vi "使用范例_单行数据存储A.vi"() -> ()   [LabVIEW 2020]
panel:
  in  "文件头（最后一个字符是换行）":string="Current Voltage\nI V\n"
  in  "存储路径":path=path "D:/"
  in  "其他说明信息":string="300K_1000Oe"
  in  "测试项目":string="IVcurve"
  in  "样品名称":string="deviceUnderTest"
  in  "是否添加时间？":bool=TRUE
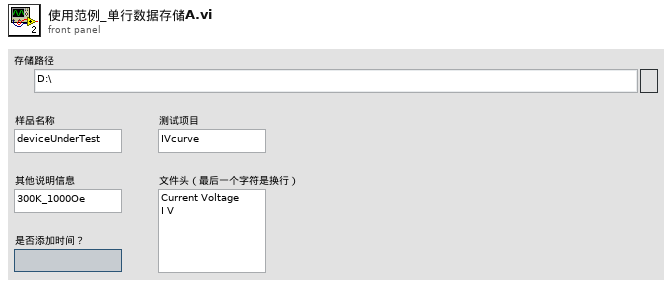
[diagram p1: front panel]
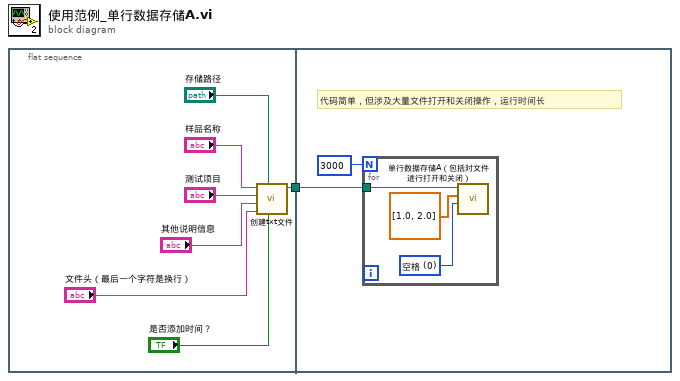
[diagram p0: block diagram]
diagram:
  n1 = flat-sequence {
    tunnel: [w8] -> w1
    tunnel: w1 -> [w9]
    frame #0 {
      n2 = call "创建txt文件.vi"("是否添加时间？"="是否添加时间？", "存储路径"="存储路径", "文件头（最后一个字符是换行）"="文件头（最后一个字符是换行）", "其他说明信息"="其他说明信息", "测试项目"="测试项目", "样品名称"="样品名称") -> ("文件路径"=w8:path)  [unwired: 5 in]
    }
    frame #1 {
      # "代码简单，但涉及大量文件打开和关闭操作，运行时间长"
      n3 = for {
        N: 3000 -> [_]
        tunnel: w9 -> [w13]
        w11 = u16 0 items=["空格", "制表符"] ("分隔符")
        n4 = call "单行数据存储A（包括对文件进行打开和关闭）.vi"("分隔符"=w11, "存储向量"=dbl[] [1.0, 2.0], "文件路径"=w13) -> ()  [unwired: 8 in]
      }
    }
  }
